vi "Hide Panel.vi"(8 "error in (no error)":errorcluster) -> (0 "error out":errorcluster)   [LabVIEW 2021, in "Master.lvlib"]
doc: "Send the Hide Panel request to the Module's Main.vi.\n_____\nBased on DQMH Project Template 6.1.0.94."
uses:
  Master.lvlib
  Hide Panel Argument--cluster.ctl
  <vilib>/DQMH Consortium/Lumos API/Libraries/SDV API/SDV API.lvlib
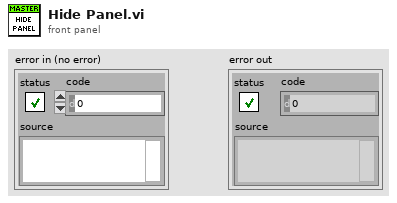
[diagram p1: front panel]
types:
  T1 = typedef "Master.lvlib/Hide Panel Argument--cluster.ctl" = cluster{"Hide Panel?":bool}
  T2 = typedef "Master.lvlib/Request Events--cluster.ctl" = cluster{"Stop Module":refnum<user-event>, "Show Panel":refnum<user-event>, "Hide Panel":refnum<user-event>, "Get Module Execution Status":refnum<user-event>, "Show Diagram":refnum<user-event>, "Slave Launch":refnum<user-event>, "Slave Stop":refnum<user-event>}
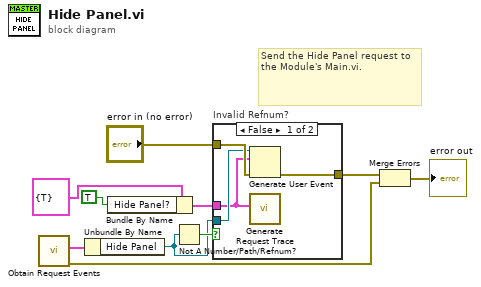
[diagram p0: block diagram]
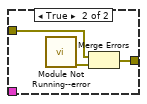
[diagram p2: hidden frame]
diagram:
  # "Send the Hide Panel request to the Module's Main.vi."
  n1 = call "Obtain Request Events.vi"() -> ("error out"=w9:errorcluster, "Master Request Events"=w8:T2)  [unwired: 10 in]
  n2 = Unbundle By Name(w8) -> ("Hide Panel"=w6:refnum<user-event>)
  n3 = Bundle By Name(cluster=T1 {"Hide Panel?"=TRUE} ("Hide Panel Argument"), "Hide Panel?"=TRUE) -> (w2:T1)
  n4 = Not A Number/Path/Refnum?(number/path/refnum=w6) -> (NaN/Path/Refnum?=w7:bool)
  n5 = case "Invalid Refnum?" shown="False" w7 {
    tunnel: "error in (no error)" -> [w14 w15]
    tunnel: [w13 w16] -> w4
    tunnel: w6 -> [w12 _]
    tunnel: w2 -> [w11 _]
    frame False {
      n6 = Generate User Event(user event=w12, event data cluster=w11, error in=w14) -> (error out=w13:errorcluster)  [unwired: 1 in, 1 out]
      n7 = call <vilib>:"Generate Request Trace.vi"("Payload"=w11) -> ()  [unwired: 10 in, 1 out]
    }
    frame True {
      n8 = call "Module Not Running--error.vi"() -> ("error out"=w17:errorcluster)  [unwired: 11 in]
      n9 = Merge Errors(w15, w17) -> (w16:errorcluster)
    }
  }
  n10 = Merge Errors(w4, w9) -> (→"error out":errorcluster)
